vi "Read.EngineData.vi"(8 "error in":errorcluster, 11 "Read in":refnum<class "Read.lvclass">) -> (0 "error out":errorcluster, 3 "Read out":refnum<class "Read.lvclass">)   [LabVIEW 2015, in "Data Access API.lvlib" / "Read.lvclass"]
uses:
  Read.lvclass
  Read.lvclass/Read.ctl
  <vilib>/NI Veristand/Custom Device API/Global Data Refs.vi
  <vilib>/NI Veristand/Custom Device API/Custom Device API.lvlib
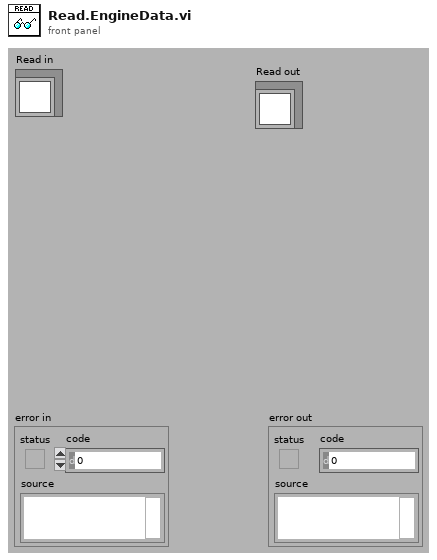
[diagram p1: front panel]
types:
  T1 = typedef "Custom Device API.lvlib/Block Data Reference.ctl" = cluster{"Data Reference":T2, "Offset":u64, "Length":u64}
  T2 = typedef "Custom Device API.lvlib/Data Reference.ctl" = i32
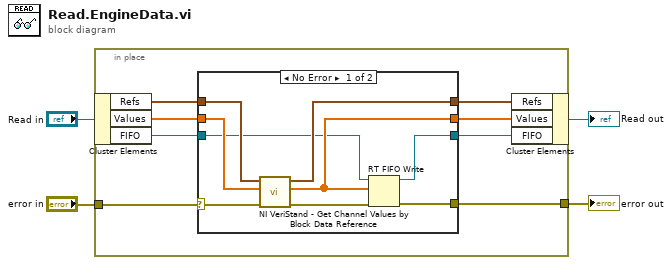
[diagram p0: block diagram]
diagram:
  n1 = in-place {
    in-place-border: [w12] -> w4
    in-place-border: "error in" -> [w9]
    n2 = in-place-cluster #1("Read in") -> ("Refs"=w11:T1[], "Values"=w8:dbl[], "FIFO"=w6:refnum<k33>)
    n3 = case shown="No Error" w9 {
      selector: w9 -> [w20 w25]
      tunnel: [w21 w25] -> w12
      tunnel: [w15 w23] -> w7
      tunnel: w11 -> [w18 w24]
      tunnel: [w17 w24] -> w10
      tunnel: w8 -> [w16 w23]
      tunnel: w6 -> [w14 w22]
      tunnel: [w13 w22] -> w5
      frame No Error {
        n4 = call <vilib>:"NI VeriStand - Get Channel Values by Block Data Reference.vi"("error in (no error)"=w20, "Values Array in"=w16, "Block Data Ref"=w18) -> ("error out"=w19:errorcluster, "Values Array out"=w15:dbl[], "Block Data Ref dup"=w17:T1[])  [unwired: 6 in]
        n5 = RT FIFO Write(0:w14, 1:w15, 3:w19) -> (8:w13:refnum<k33>, 11:w21:errorcluster)  [unwired: 2 in, 2 out]
      }
      frame Error {
      }
    }
    n6 = in-place-cluster #1("Refs"=w10, "Values"=w7, "FIFO"=w5) -> (→"Read out":refnum<class "Read.lvclass">)
  }
  "error out" <- w4
